vi "ReadWriteDataLoop.vi"(10 "Clock":i64=100) -> ()   [LabVIEW 2011]
uses:
  <vilib>/Platform/TimedLoop/XDataNode/timing_clust.ctl
  <vilib>/Platform/TimedLoop/XDataNode/nitl_modes.ctl
  <vilib>/Platform/TimedLoop/XDataNode/wakeup.ctl
  GlobalVariables.vi
  DS/DSRead int16.vi
  DS/DSRead uint8.vi
  DS/DSRead bool.vi
  DS/DSRead uint32.vi
  <vilib>/Platform/TimedLoop/XDataNode/XDataNode.xnode
  <vilib>/Platform/TimedLoop/XDataNode/XDNodeRunTimeDep.lvlib
  DS/DSWrite uint32.vi
panel:
  in  "CloseVi?":bool
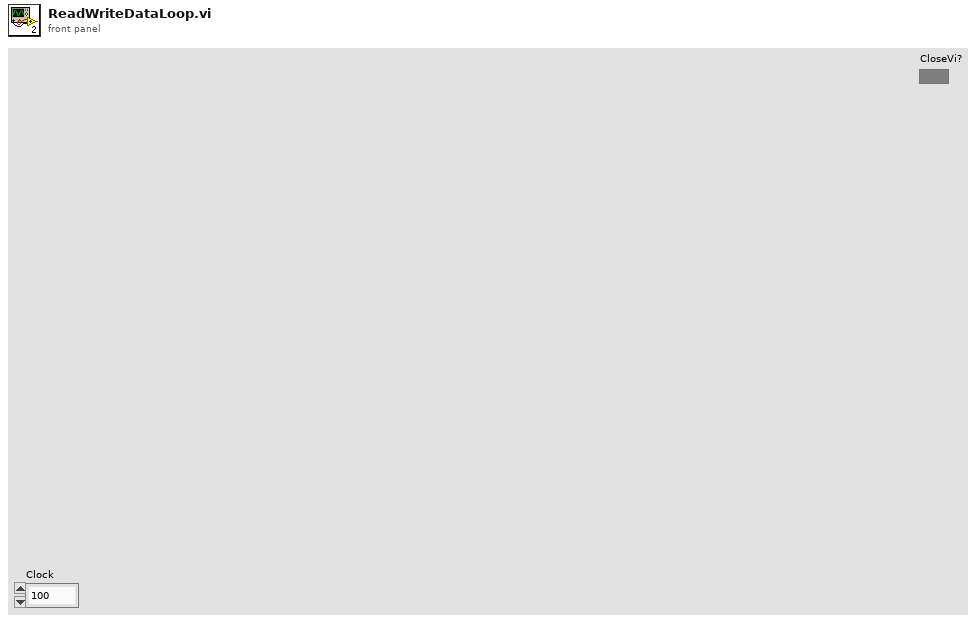
[diagram p1: front panel]
types:
  T1 = enum16{"Read", "Write", "ReadWrite", "BufferedRead", "BufferedReadWrite"}
  T2 = enum16{"OPC Server", "Global", "Dnet1", "Dnet2", "Dnet3", "Ain1", "Ain2", "Aout1", "Din1", "Din2", "Dout1"}
  T3 = typedef "XDNodeRunTimeDep.lvlib/timing_clust.ctl" = cluster{"Expected End [f-1]":u64, "Actual End [f-1]":u64, "Finished Late? [f-1]":bool, "Expected End [i-1]":u64, "Actual End [i-1]":u64, "Finished Late? [i-1]":bool, "Expected Start [i]":u64, "Actual Start [i]":u64, "Expected Start [f]":u64, "Actual Start [f]":u64, "Source Name":string, "Structure Name":string, "Period":i64, "Deadline":i64, "Offset":i64, "Start":i64, "Priority":i32, "Timeout":i32, "Mode":T4, "Wakeup Reason":T5, "Error":errorcluster, "Source Type":string, "Secondary Source Type":string, "Global End Time":u64, "Global Start Time":u64, "Frame Duration":u64, "Iteration Duration":u64, "Assigned CPU":i32, "I/O Scan Engine Mode":u32}
  T4 = typedef "XDNodeRunTimeDep.lvlib/nitl_modes.ctl" = enum32{"No Change", "Process missed periods, maintain original phase", "Discard missed periods, maintain original phase", "Process missed periods, ignore original phase", "Discard missed periods, ignore original phase"}
  T5 = typedef "XDNodeRunTimeDep.lvlib/wakeup.ctl" = enum32{"Normal", "Aborted", "Asynchronous wakeup", "Timing source error", "Timed loop error", "Timeout"}
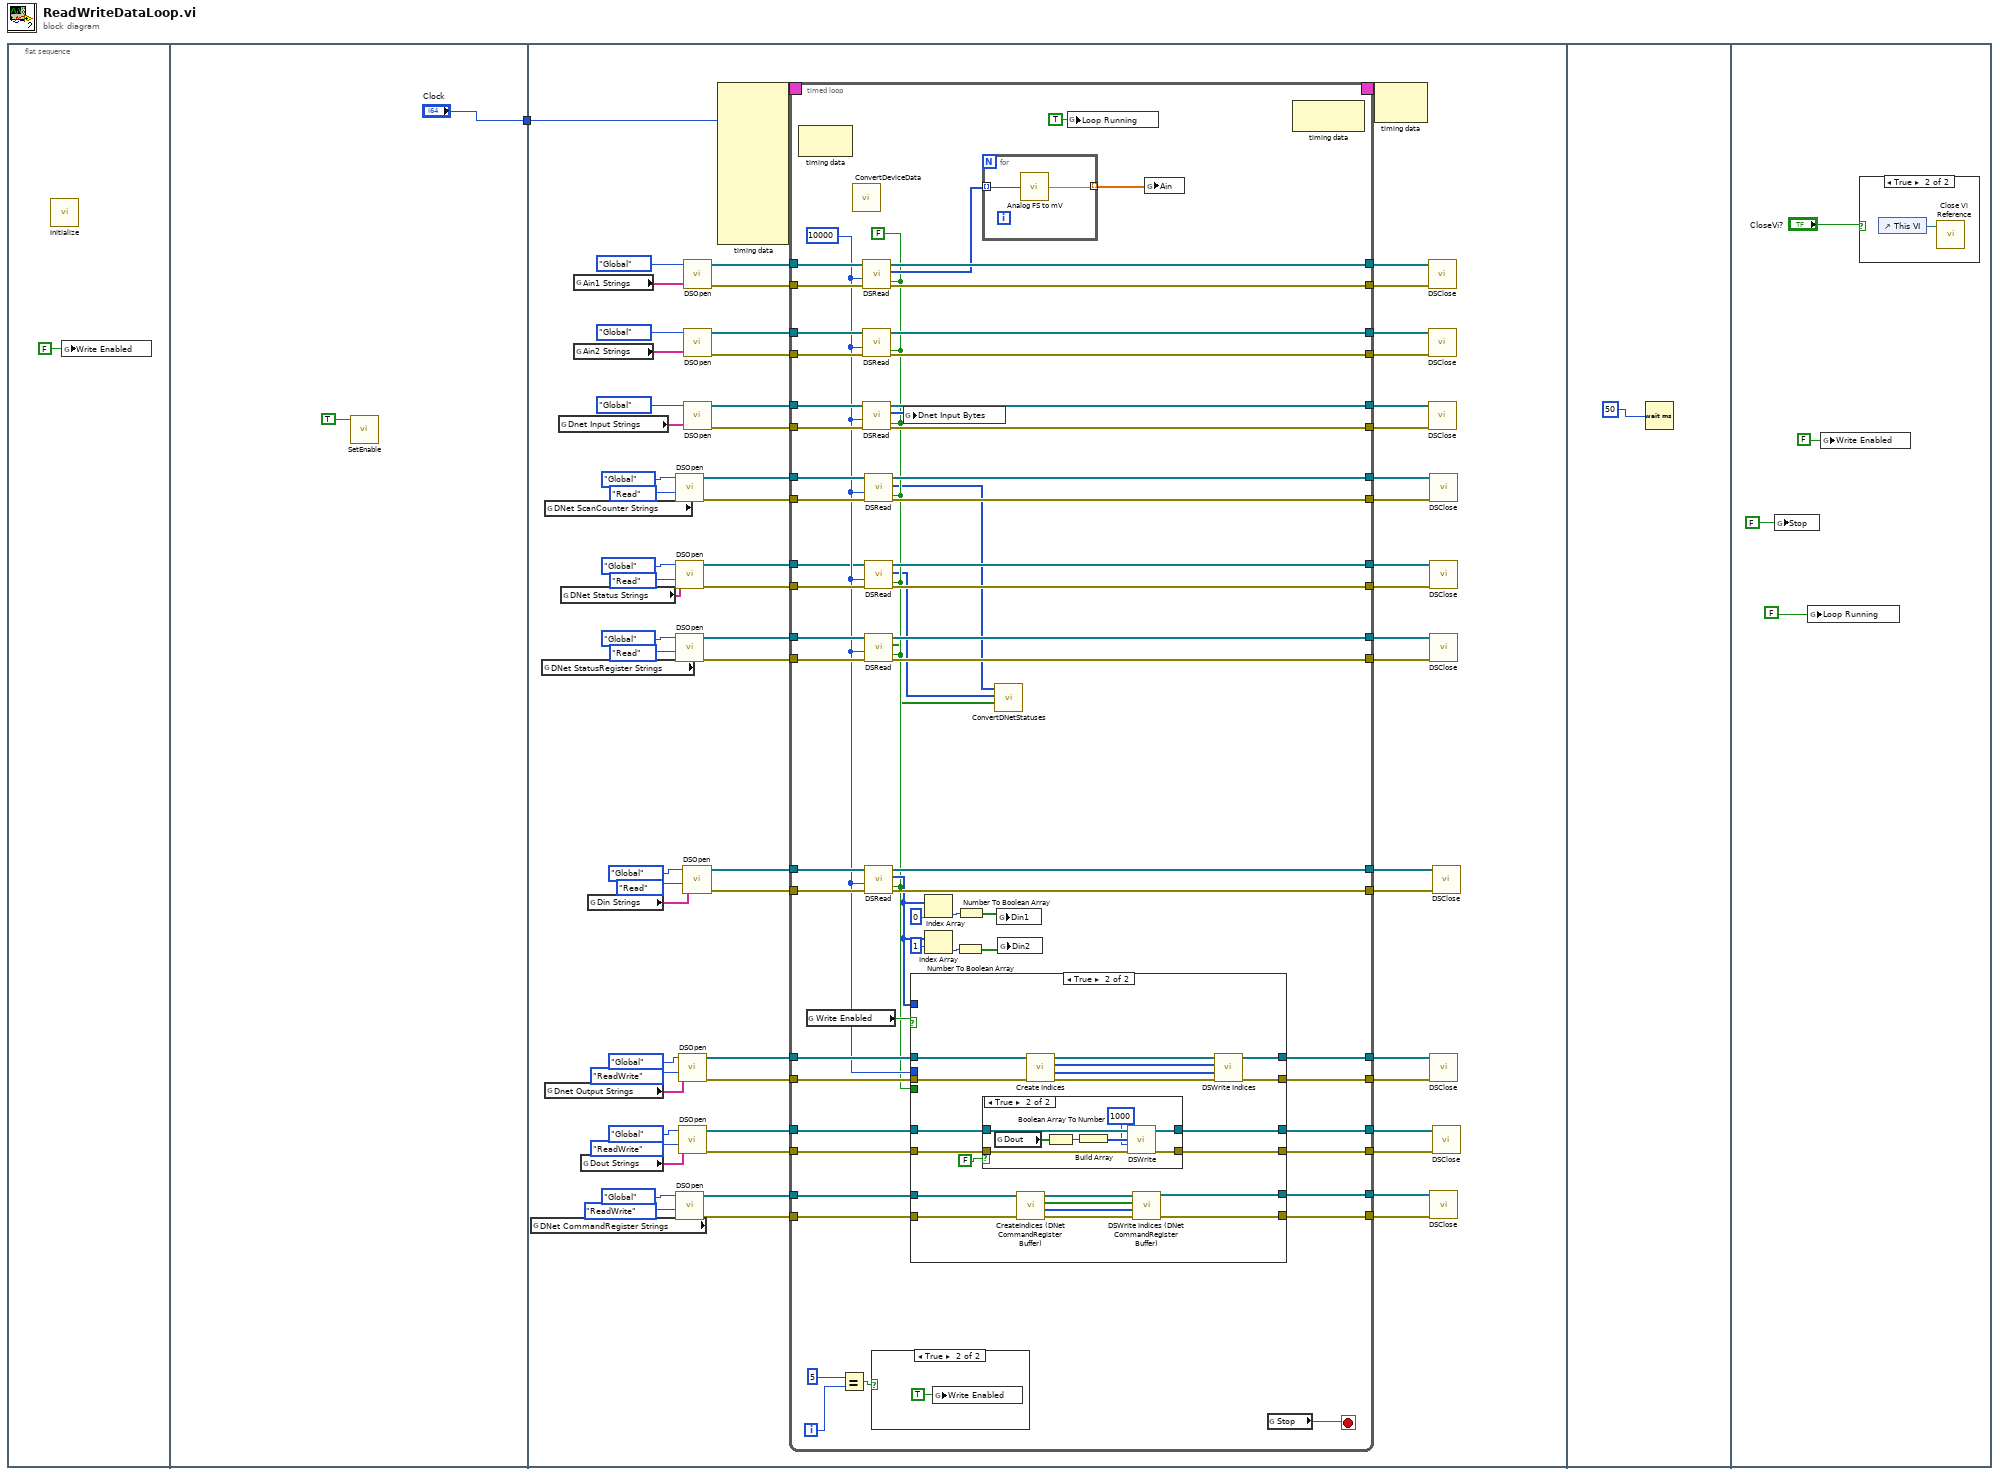
[diagram p0: block diagram]
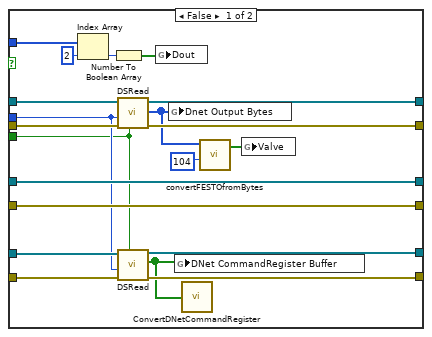
[diagram p3: hidden frame]
diagram:
  n1 = flat-sequence {
    tunnel: ["Clock"] -> w1
    tunnel: w1 -> [w33]
    frame #0 {
      n2 = call "Initialize.vi"() -> ()  [unwired: 12 in]
      n3 = global write "GlobalVariables.vi" "Write Enabled"(FALSE ("Reinitialize?")) -> ()
    }
    frame #1 {
      n4 = call "SetEnable.vi"("Enabled/Disable"=TRUE) -> ()  [unwired: 11 in]
    }
    frame #2 {
      n5 = global read "GlobalVariables.vi" "DNet CommandRegister Strings"() -> (w22:string[])
      n6 = global read "GlobalVariables.vi" "DNet StatusRegister Strings"() -> (w25:string[])
      n7 = global read "GlobalVariables.vi" "DNet ScanCounter Strings"() -> (w31:string[])
      n8 = global read "GlobalVariables.vi" "Dnet Output Strings"() -> (w53:string[])
      n9 = global read "GlobalVariables.vi" "Dnet Input Strings"() -> (w59:string[])
      n10 = global read "GlobalVariables.vi" "DNet Status Strings"() -> (w28:string[])
      n11 = global read "GlobalVariables.vi" "Ain1 Strings"() -> (w71:string[])
      n12 = global read "GlobalVariables.vi" "Ain2 Strings"() -> (w65:string[])
      n13 = global read "GlobalVariables.vi" "Dout Strings"() -> (w39:string[])
      n14 = global read "GlobalVariables.vi" "Din Strings"() -> (w46:string[])
      n15 = call "DSOpen.vi"("Array"=w31, "mode"=T1."Read", "Slot"=T2."Global") -> ("error Out"=w20:errorcluster[], "connection out"=w19:refnum<k13>[])  [unwired: 7 in]
      n16 = call "DSOpen.vi"("Array"=w28, "mode"=T1."Read", "Slot"=T2."Global") -> ("error Out"=w16:errorcluster[], "connection out"=w5:refnum<k13>[])  [unwired: 7 in]
      n17 = call "DSOpen.vi"("Array"=w25, "mode"=T1."Read", "Slot"=T2."Global") -> ("error Out"=w13:errorcluster[], "connection out"=w12:refnum<k13>[])  [unwired: 7 in]
      n18 = call "DSOpen.vi"("Array"=w22, "mode"=T1."ReadWrite", "Slot"=T2."Global") -> ("error Out"=w15:errorcluster[], "connection out"=w14:refnum<k13>[])  [unwired: 7 in]
      n19 = call "DSOpen.vi"("Array"=w53, "mode"=T1."ReadWrite", "Slot"=T2."Global") -> ("error Out"=w51:errorcluster[], "connection out"=w50:refnum<k13>[])  [unwired: 7 in]
      n20 = call "DSOpen.vi"("Array"=w39, "mode"=T1."ReadWrite", "Slot"=T2."Global") -> ("error Out"=w37:errorcluster[], "connection out"=w36:refnum<k13>[])  [unwired: 7 in]
      n21 = call "DSOpen.vi"("Array"=w46, "mode"=T1."Read", "Slot"=T2."Global") -> ("error Out"=w44:errorcluster[], "connection out"=w43:refnum<k13>[])  [unwired: 7 in]
      n22 = call "DSOpen.vi"("Array"=w71, "Slot"=T2."Global") -> ("error Out"=w70:errorcluster[], "connection out"=w69:refnum<k13>[])  [unwired: 8 in]
      n23 = call "DSOpen.vi"("Array"=w65, "Slot"=T2."Global") -> ("error Out"=w64:errorcluster[], "connection out"=w63:refnum<k13>[])  [unwired: 8 in]
      n24 = call "DSOpen.vi"("Array"=w59, "Slot"=T2."Global") -> ("error Out"=w57:errorcluster[], "connection out"=w58:refnum<k13>[])  [unwired: 8 in]
      n25 = node-c288(w33) -> (w74:T3)  [unwired: 9 in]
      n26 = timed-loop {
        tunnel: w70 -> [w134]
        tunnel: w69 -> [w133]
        tunnel: [w131] -> w68
        tunnel: [w130] -> w67
        tunnel: w64 -> [w128]
        tunnel: w63 -> [w127]
        tunnel: [w126] -> w62
        tunnel: [w125] -> w61
        tunnel: w58 -> [w124]
        tunnel: w57 -> [w123]
        tunnel: [w122] -> w55
        tunnel: [w121] -> w56
        timing: w74 -> [_]
        timing-out: [_] -> w73
        tunnel: w51 -> [w120]
        tunnel: w50 -> [w119]
        tunnel: [w118] -> w49
        tunnel: [w117] -> w48
        tunnel: w44 -> [w115]
        tunnel: w43 -> [w114]
        tunnel: [w107] -> w42
        tunnel: [w106] -> w41
        tunnel: w37 -> [w105]
        tunnel: w36 -> [w104]
        tunnel: [w103] -> w35
        tunnel: [w102] -> w34
        tunnel: w20 -> [w99]
        tunnel: w19 -> [w98]
        tunnel: [w97] -> w18
        tunnel: [w96] -> w17
        tunnel: w16 -> [w95]
        tunnel: w15 -> [w88]
        tunnel: w14 -> [w87]
        tunnel: w13 -> [w94]
        tunnel: w12 -> [w93]
        tunnel: [w86] -> w11
        tunnel: [w85] -> w10
        tunnel: [w92] -> w9
        tunnel: [w91] -> w8
        tunnel: [w90] -> w7
        tunnel: [w89] -> w6
        tunnel: w5 -> [w79]
        i -> [w76]
        stop <- w135 stop-if-true
        w84 = 10000 ("ms timeout (10000)")
        w83 = FALSE ("wait for updated value (T)")
        n27 = node-c288() -> ()  [unwired: 1 in, 1 out]
        n28 = global read "GlobalVariables.vi" "Write Enabled"() -> (w116:bool)
        n29 = Equal?(x=5, y=w76) -> (x = y?=w77:bool)
        n30 = call "ConvertDeviceData.vi"() -> ()  [unwired: 12 in]
        n31 = call-poly "DSRead.vi"("wait for updated value (T)"=w83, "error in"=w134, "ms timeout (10000)"=w84, "connection in"=w133) -> ("error out"=w130:errorcluster[], "data"=w129:i16[], "connection out"=w131:refnum<k13>[])  [unwired: 5 in]
        n32 = call-poly "DSRead.vi"("wait for updated value (T)"=w83, "error in"=w128, "ms timeout (10000)"=w84, "connection in"=w127) -> ("error out"=w126:errorcluster[], "connection out"=w125:refnum<k13>[])  [unwired: 5 in, 1 out]
        n33 = call-poly "DSRead.vi"("wait for updated value (T)"=w83, "error in"=w123, "ms timeout (10000)"=w84, "connection in"=w124) -> ("error out"=w121:errorcluster[], "data"=w101:u8[], "connection out"=w122:refnum<k13>[])  [unwired: 5 in]
        n34 = call-poly "DSRead.vi"("wait for updated value (T)"=w83, "error in"=w99, "ms timeout (10000)"=w84, "connection in"=w98) -> ("error out"=w97:errorcluster[], "data"=w82:u32[], "connection out"=w96:refnum<k13>[])  [unwired: 5 in]
        n35 = call-poly "DSRead.vi"("wait for updated value (T)"=w83, "error in"=w95, "ms timeout (10000)"=w84, "connection in"=w79) -> ("error out"=w90:errorcluster[], "data"=w80:u8[], "connection out"=w89:refnum<k13>[])  [unwired: 5 in]
        n36 = call-poly "DSRead.vi"("wait for updated value (T)"=w83, "error in"=w94, "ms timeout (10000)"=w84, "connection in"=w93) -> ("error out"=w92:errorcluster[], "data"=w81:bool[], "connection out"=w91:refnum<k13>[])  [unwired: 5 in]
        n37 = call-poly "DSRead.vi"("wait for updated value (T)"=w83, "error in"=w115, "ms timeout (10000)"=w84, "connection in"=w114) -> ("error out"=w106:errorcluster[], "data"=w100:u32[], "connection out"=w107:refnum<k13>[])  [unwired: 5 in]
        n38 = case shown="True" w77 {
          frame False {
          }
          frame True {
            n39 = global write "GlobalVariables.vi" "Write Enabled"(TRUE ("Write Enabled")) -> ()
          }
        }
        n40 = global write "GlobalVariables.vi" "Dnet Input Bytes"(w101) -> ()
        n41 = case shown="True" w116 {
          tunnel: w120 -> [w156 w173]
          tunnel: w119 -> [w155 w172]
          tunnel: [w154 w170] -> w118
          tunnel: [w153 w171] -> w117
          tunnel: w105 -> [w151 w174]
          tunnel: w104 -> [w152 w175]
          tunnel: [w151 w177] -> w103
          tunnel: [w152 w176] -> w102
          tunnel: w100 -> [w144 _]
          tunnel: w88 -> [w143 w163]
          tunnel: w87 -> [w142 w164]
          tunnel: [w141 w161] -> w86
          tunnel: [w140 w160] -> w85
          tunnel: w84 -> [w139 _]
          tunnel: w83 -> [w138 _]
          frame False {
            n42 = Index Array(array=w144, index=2) -> (element=w145:u32)
            n43 = Number To Boolean Array(number=w145) -> (Boolean array=w149:bool[])
            n44 = call-poly "DSRead.vi"("wait for updated value (T)"=w138, "error in"=w156, "ms timeout (10000)"=w139, "connection in"=w155) -> ("error out"=w154:errorcluster[], "data"=w148:u8[], "connection out"=w153:refnum<k13>[])  [unwired: 5 in]
            n45 = call-poly "DSRead.vi"("wait for updated value (T)"=w138, "error in"=w143, "ms timeout (10000)"=w139, "connection in"=w142) -> ("error out"=w141:errorcluster[], "data"=w137:bool[], "connection out"=w140:refnum<k13>[])  [unwired: 5 in]
            n46 = global write "GlobalVariables.vi" "Dout"(w149) -> ()
            n47 = global write "GlobalVariables.vi" "Dnet Output Bytes"(w148) -> ()
            n48 = global write "GlobalVariables.vi" "DNet CommandRegister Buffer"(w137) -> ()
            n49 = call "ConvertDNetCommandRegister.vi"("CommandRegisterBit Array"=w137) -> ()  [unwired: 1 in]
            n50 = call "convertFESTOfromBytes.vi"("Start Byte"=104, "Bytes"=w148) -> ("data"=w146:bool[])  [unwired: 9 in]
            n51 = global write "GlobalVariables.vi" "Valve"(w146) -> ()
          }
          frame True {
            n52 = case shown="True" FALSE {
              tunnel: [w179 w187] -> w177
              tunnel: [w178 w186] -> w176
              tunnel: w175 -> [w178 w185]
              tunnel: w174 -> [w179 w184]
              frame False {
              }
              frame True {
                n53 = global read "GlobalVariables.vi" "Dout"() -> (w183:bool[])
                n54 = Boolean Array To Number(Boolean array=w183) -> (number=w182:u32)
                n55 = Build Array(w182) -> (w181:u32[])
                n56 = call-poly "DSWrite.vi"("error in"=w184, "ms timeout (10000)"=1000, "data"=w181, "connection in"=w185) -> ("error out"=w187:errorcluster[], "connection out"=w186:refnum<k13>[])  [unwired: 6 in]
              }
            }
            n57 = call "CreateIndices (DNet CommandRegister Buffer).vi"("error in"=w163, "connection in"=w164) -> ("error out"=w162:errorcluster[], "Indices"=w157:i32[], "DNet CommandRegister Buffer"=w158:bool[], "connection out"=w159:refnum<k13>[])  [unwired: 6 in]
            n58 = call "Create Indices.vi"("error in"=w173, "connection in"=w172) -> ("error out"=w169:errorcluster[], "Indices"=w167:i32[], "Dnet Output Bytes"=w165:u8[], "connection out"=w168:refnum<k13>[])  [unwired: 6 in]
            n59 = call "DSWrite Indices (DNet CommandRegister Buffer).vi"("error in"=w162, "Indices"=w157, "data"=w158, "connection in"=w159) -> ("error out"=w161:errorcluster[], "connection out"=w160:refnum<k13>[])  [unwired: 6 in]
            n60 = call "DSWrite Indices.vi"("error in"=w169, "Indices"=w167, "data"=w165, "connection in"=w168) -> ("error out"=w170:errorcluster[], "connection out"=w171:refnum<k13>[])  [unwired: 6 in]
          }
        }
        n61 = Index Array(array=w100, index=0) -> (element=w110:u32)
        n62 = Index Array(array=w100, index=1) -> (element=w111:u32)
        n63 = Number To Boolean Array(number=w111) -> (Boolean array=w109:bool[])
        n64 = Number To Boolean Array(number=w110) -> (Boolean array=w108:bool[])
        n65 = for {
          tunnel: w129 -> [w191] mode=indexing
          tunnel: [w190] -> w132 mode=indexing
          n66 = call "Analog FS to mV.vi"("input"=w191) -> ("output"=w190:dbl)
        }
        n67 = call "ConvertDNetStatuses.vi"("StatusRegister"=w81, "Status Array"=w80, "ScanCounter Array"=w82) -> ()  [unwired: 9 in]
        n68 = global write "GlobalVariables.vi" "Din1"(w108) -> ()
        n69 = global write "GlobalVariables.vi" "Din2"(w109) -> ()
        n70 = global write "GlobalVariables.vi" "Loop Running"(TRUE ("Loop Started")) -> ()
        n71 = global write "GlobalVariables.vi" "Ain"(w132) -> ()
        n72 = global read "GlobalVariables.vi" "Stop"() -> (w135:bool)
        n73 = node-c288() -> ()  [unwired: 1 in, 1 out]
      }
      n74 = node-c288(w73) -> ()  [unwired: 1 out]
      n75 = call "DSClose.vi"("error in (no error)"=w67, "connection id"=w68) -> ()  [unwired: 10 in]
      n76 = call "DSClose.vi"("error in (no error)"=w62, "connection id"=w61) -> ()  [unwired: 10 in]
      n77 = call "DSClose.vi"("error in (no error)"=w56, "connection id"=w55) -> ()  [unwired: 10 in]
      n78 = call "DSClose.vi"("error in (no error)"=w18, "connection id"=w17) -> ()  [unwired: 10 in]
      n79 = call "DSClose.vi"("error in (no error)"=w7, "connection id"=w6) -> ()  [unwired: 10 in]
      n80 = call "DSClose.vi"("error in (no error)"=w9, "connection id"=w8) -> ()  [unwired: 10 in]
      n81 = call "DSClose.vi"("error in (no error)"=w49, "connection id"=w48) -> ()  [unwired: 10 in]
      n82 = call "DSClose.vi"("error in (no error)"=w11, "connection id"=w10) -> ()  [unwired: 10 in]
      n83 = call "DSClose.vi"("error in (no error)"=w41, "connection id"=w42) -> ()  [unwired: 10 in]
      n84 = call "DSClose.vi"("error in (no error)"=w35, "connection id"=w34) -> ()  [unwired: 10 in]
    }
    frame #3 {
      n85 = Wait (ms)(milliseconds to wait=50) -> ()  [unwired: 1 out]
    }
    frame #4 {
      n86 = global write "GlobalVariables.vi" "Stop"(FALSE ("stop")) -> ()
      n87 = global write "GlobalVariables.vi" "Loop Running"(FALSE ("stop")) -> ()
      n88 = global write "GlobalVariables.vi" "Write Enabled"(FALSE ("Reinitialize?")) -> ()
      n89 = case shown="True" "CloseVi?" {
        frame False {
        }
        frame True {
          n90 = control-ref of="This VI"() -> (w201:refnum<vi>)
          n91 = call "Close Vi Reference.vi"("reference"=w201) -> ()  [unwired: 9 in, 2 out]
        }
      }
    }
  }
